vi "Control_de-activate.vi"(0 "Boolean":bool=TRUE, 1 "reference":refnum<vi>) -> ()   [LabVIEW 2015]
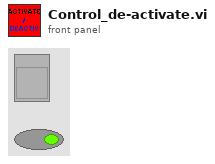
[diagram p1: front panel]
types:
  T1 = enum8{"Enabled", "Disabled", "Disabled and Grayed Out"}
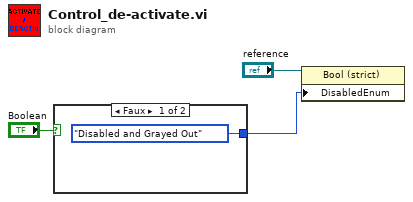
[diagram p0: block diagram]
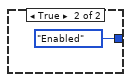
[diagram p2: hidden frame]
diagram:
  n1 = case shown="Faux" "Boolean" {
    tunnel: [T1."Disabled and Grayed Out" ("Disabled") T1."Enabled" ("Disabled")] -> w3
    frame False {
    }
    frame True {
    }
  }
  n2 = property class="Bool (strict)"(reference="reference", "DisabledEnum"=w3) -> ()  [unwired: 1 in, 2 out]
